vi "Query Max Voltage Level.vi"(8 "error in (no error)":errorcluster, 9 "current limit (0.0 Amps)":dbl[unit] format="%^.2e", 10 "channel name (\"CHANNEL1\")":string="CHANNEL1", 11 "CS++DCPwr in":refnum<class "CS++DCPwr.lvclass">) -> (0 "error out":errorcluster, 2 "max voltage level":dbl[unit] format="%^.2e", 3 "CS++DCPwr out":refnum<class "CS++DCPwr.lvclass">)   [LabVIEW 2013, in "CS++DCPwr.lvlib" / "CS++DCPwr.lvclass"]
doc: "This VI returns the maximum programmable voltage level that the power supply accepts for a particular current limit on a channel for the output range to which the power supply is currently configured."
uses:
  CS++DCPwr.lvclass
  Core/Classes/CS++ProcessVariables/ProcessVariable/PV.lvclass
  Core/Classes/CS++ProcessVariables/ProcessVariable/PV.lvclass/PV.ctl
  CS++DCPwr.lvclass/CS++DCPwr.ctl
  Core/Classes/CS++ProcessVariables/PVConnection/PVConnection.lvclass
  Core/Classes/CS++ProcessVariables/ProcessVariable/Write Data.vi
  Core/Classes/CS++ProcessVariables/ProcessVariable/Write Timestamp.vi
  Core/Classes/CS++ProcessVariables/ProcessVariable/Write Quality.vi
  Core/Classes/CS++ProcessVariables/ProcessVariable/Write status.vi
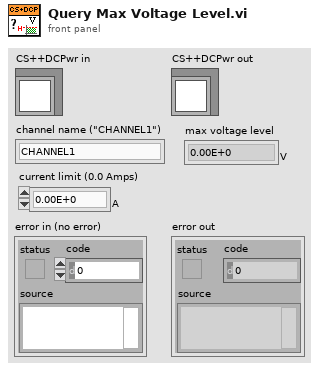
[diagram p1: front panel]
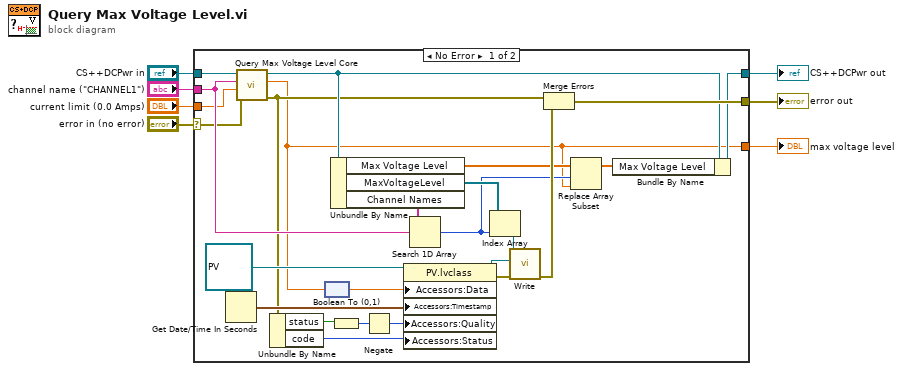
[diagram p0: block diagram]
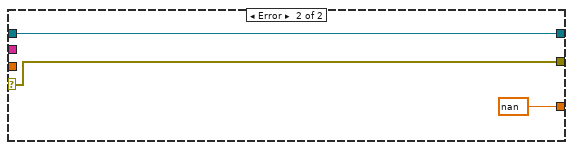
[diagram p2: hidden frame]
diagram:
  n1 = case shown="No Error" "error in (no error)" {
    selector: "error in (no error)" -> [w12 w34]
    tunnel: "CS++DCPwr in" -> [w15 w35]
    tunnel: "current limit (0.0 Amps)" -> [w13 _]
    tunnel: "channel name (\"CHANNEL1\")" -> [w14 _]
    tunnel: [w20 w34] -> w5
    tunnel: [w19 w35] -> w7
    tunnel: [w9 dbl[unit] nan ("max current limit")] -> w6
    frame No Error {
      n2 = Get Date/Time In Seconds() -> (seconds since 1Jan1904=w32:timestamp)
      n3 = call-dynamic "Query Max Voltage Level Core.vi"("error in (no error)"=w12, "current limit (0.0 Amps)"=w13, "channel name (\"CHANNEL1\")"=w14, "CS++DCPwr in"=w15) -> ("error out"=w10:errorcluster, "max voltage level"=w9:dbl[unit], "CS++DCPwr out"=w11:refnum<class "CS++DCPwr.lvclass">)  [unwired: 5 in]
      n4 = Unbundle By Name(w10) -> ("status"=w24:bool, "code"=w22:i32)
      n5 = node(w9) -> (w8:dbl)
      n6 = Unbundle By Name(w11) -> ("Max Voltage Level"=w18:dbl[unit][], "MaxVoltageLevel"=w27:refnum<class "PVConnection.lvclass">[], "Channel Names"=w28:string[])
      n7 = Boolean To (0,1)(Boolean=w24) -> (0, 1=w23:i16)
      n8 = Negate(x=w23) -> (-x=w21:i16)
      n9 = property class="PV.lvclass"(reference=refnum<class "PV.lvclass"> refnum ("PV"), "Accessors:Data"=w8, "Accessors:Timestamp"=w32, "Accessors:Quality"=w21, "Accessors:Status"=w22) -> (reference out=w29:refnum<class "PV.lvclass">, error out=w30:errorcluster)  [unwired: 1 in]
      n10 = Search 1D Array(1D array=w28, element=w14) -> (index of element=w16:i32)  [unwired: 1 in]
      n11 = Index Array(array=w27, index=w16) -> (element=w26:refnum<class "PVConnection.lvclass">)
      n12 = call-dynamic "Write.vi"("error in (no error)"=w30, "PV"=w29, "PVConnection in"=w26) -> ("error out"=w25:errorcluster)  [unwired: 7 in, 1 out]
      n13 = Merge Errors(w10, w25) -> (w20:errorcluster)
      n14 = Replace Array Subset(array=w18, new element=w9, index=w16) -> (w17:dbl[unit][])
      n15 = Bundle By Name(cluster=w11, "Max Voltage Level"=w17) -> (w19:refnum<class "CS++DCPwr.lvclass">)
    }
    frame Error {
    }
  }
  "error out" <- w5
  "CS++DCPwr out" <- w7
  "max voltage level" <- w6
